vi "Main.vi"() -> ()   [LabVIEW 2014]
uses:
  Event_class/EventMsg.lvclass
  SubPanel/SubPanelModule.lvlib
panel:
  in  "Open Button":bool
  out "data":string
  in  "String":string
  in  "stop":bool
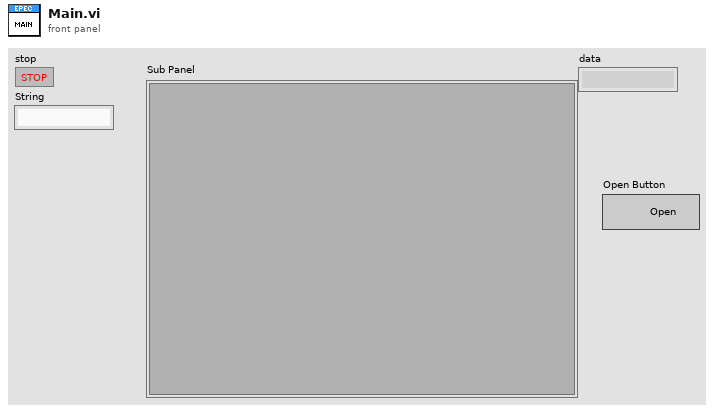
[diagram p1: front panel]
types:
  T1 = cluster{"EventClass":cluster{"object out":refnum<class "EventMsg.lvclass">}, "SubPanelData":cluster{"SubPanelPath":path, "SubPanelsVis":string[], "SubP_VIsPathList":path[], "VisRefs":refnum<vi>[]}}
  T2 = cluster{"object out":refnum<class "EventMsg.lvclass">}
  T3 = cluster{"SubPanelPath":path, "SubPanelsVis":string[], "SubP_VIsPathList":path[], "VisRefs":refnum<vi>[]}
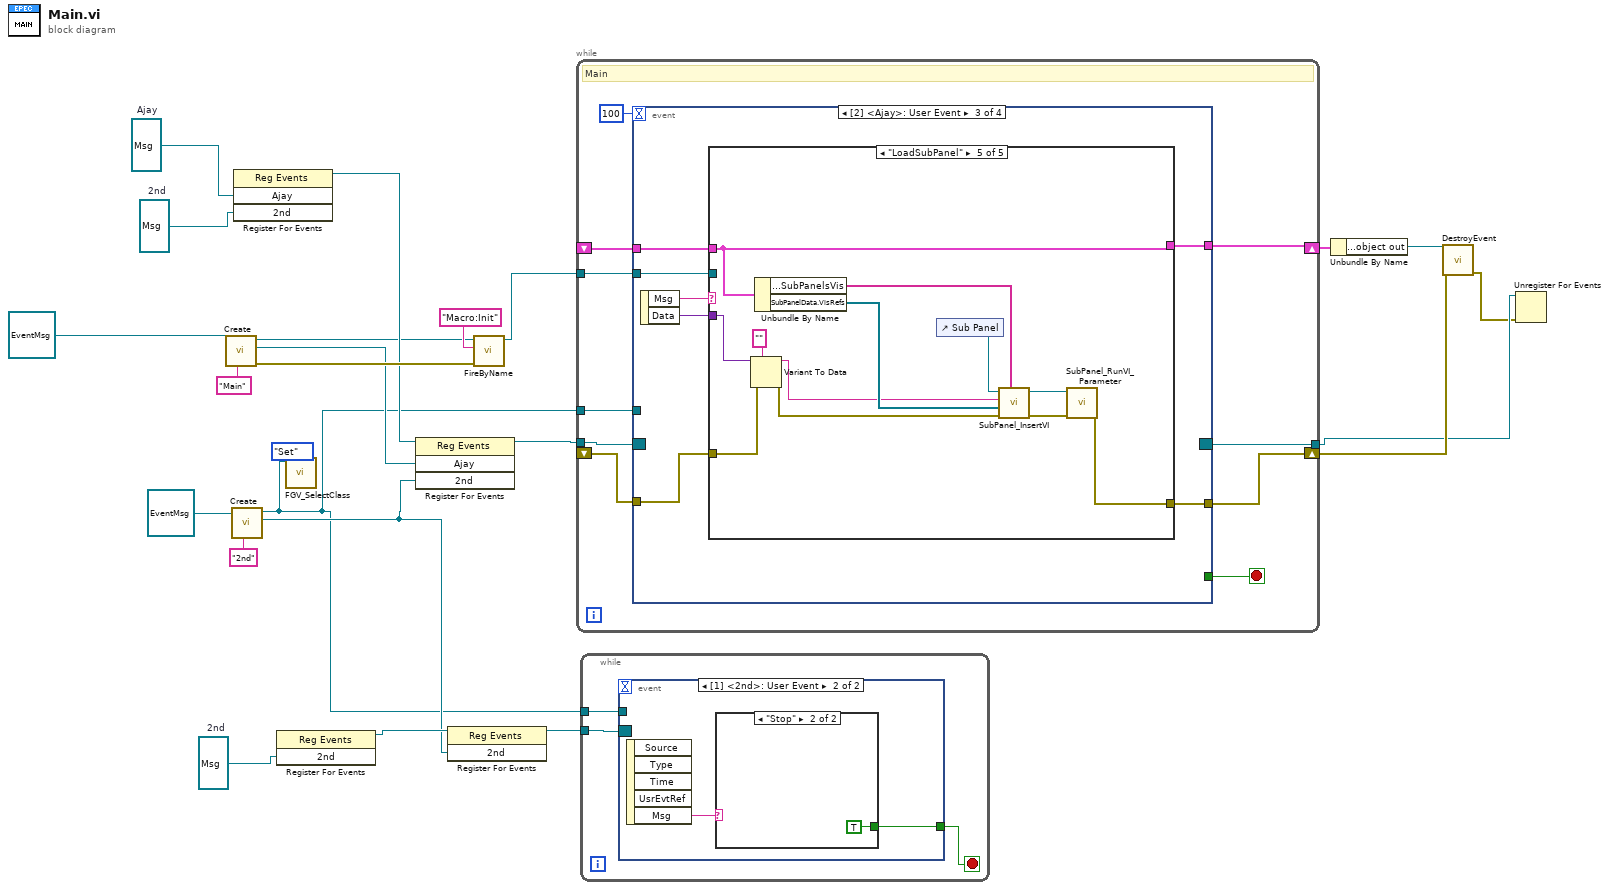
[diagram p0: block diagram]
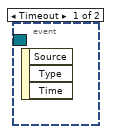
[diagram p2: hidden frame]
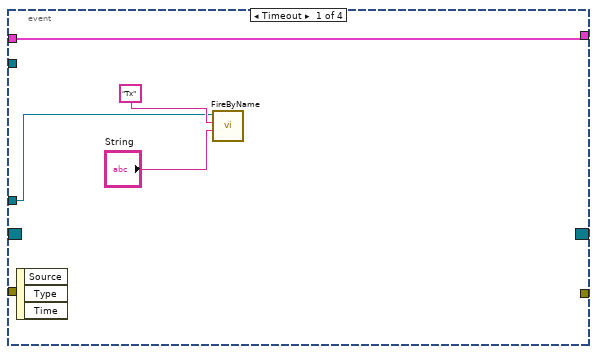
[diagram p4: hidden frame]
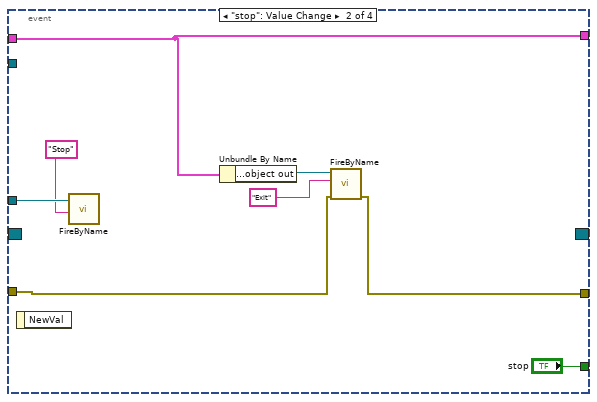
[diagram p5: hidden frame]
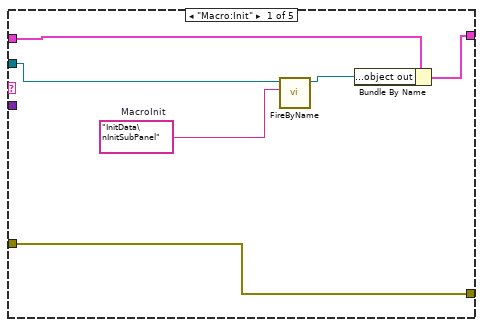
[diagram p6: hidden frame]
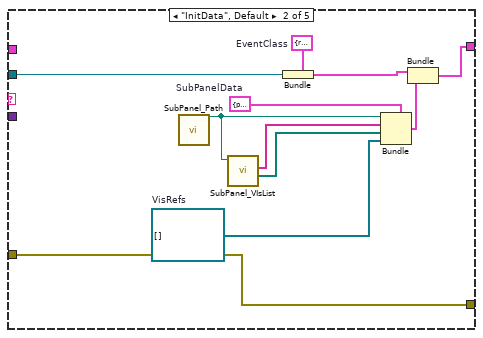
[diagram p7: hidden frame]
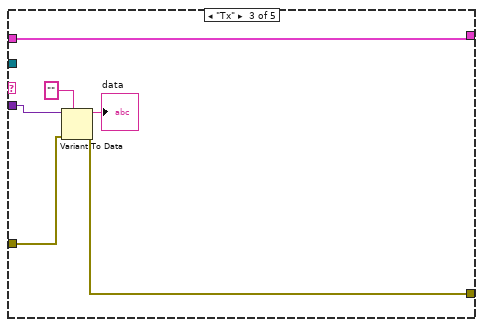
[diagram p8: hidden frame]
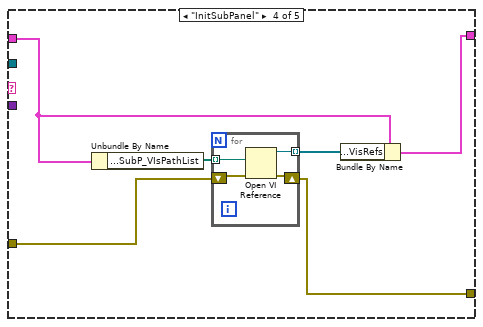
[diagram p9: hidden frame]
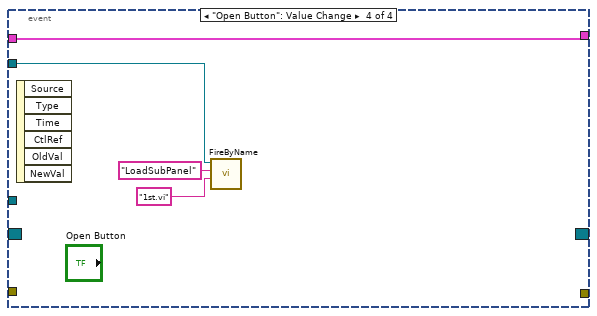
[diagram p10: hidden frame]
diagram:
  w9 = refnum<user-event> refnum  # 2nd
  w12 = refnum<user-event> refnum  # 2nd
  w17 = refnum<user-event> refnum  # Ajay
  n1 = call-dynamic "Create.vi"("Name"="Main", "object in"=refnum<class "EventMsg.lvclass"> refnum) -> ("error out"=w18:errorcluster, "user event out"=w15:refnum<user-event>, "object out"=w2:refnum<class "EventMsg.lvclass">)  [unwired: 7 in]
  n2 = call-dynamic "Create.vi"("Name"="2nd", "object in"=refnum<class "EventMsg.lvclass"> refnum) -> ("user event out"=w8:refnum<user-event>, "object out"=w1:refnum<class "EventMsg.lvclass">)  [unwired: 7 in, 1 out]
  n3 = register-events(w17, w12) -> (reference out=w16:refnum<event-registration>)  [unwired: 2 in, 1 out]
  n4 = register-events(w9) -> (reference out=w10:refnum<event-registration>)  [unwired: 2 in, 1 out]
  n5 = call "FGV_SelectClass.vi"("Action"=enum16{"Set", "Get"}."Set", "EventMsg.lvclass"=w1) -> ()  [unwired: 9 in, 1 out]
  n6 = register-events(reference=w16, w15, w8) -> (reference out=w14:refnum<event-registration>)  [unwired: 1 in, 1 out]
  n7 = register-events(reference=w10, w8) -> (reference out=w11:refnum<event-registration>)  [unwired: 1 in, 1 out]
  n8 = call-dynamic "FireByName.vi"("error in (no error)"=w18, "Msg"="Macro:Init", "object in"=w2) -> ("object out"=w22:refnum<class "EventMsg.lvclass">)  [unwired: 7 in, 1 out]
  n9 = while {
    shift-right: [w32] -> w19
    shift-left: _ -> [w33]
    shift-right: [w31] -> w21
    shift-left: _ -> [w30]
    tunnel: w22 -> [w29]
    tunnel: [w28] -> w5
    tunnel: w14 -> [w27]
    tunnel: w1 -> [w26]
    stop <- w34 stop-if-true
    # "Main"
    n10 = event shown="[2] <Ajay>: User Event" {
      selector: w27 -> [_ _ _ _]
      dyn-events: [_ _ _ _] -> w28
      timeout: 100 -> [_ _ _ _]
      tunnel: [_ "stop" _ _] -> w34
      tunnel: w33 -> [_ w43 w51 _]
      tunnel: [_ w42 w50 _] -> w32
      tunnel: [w38 w41 w49 w102] -> w31
      tunnel: w30 -> [w38 w41 w48 w102]
      tunnel: w29 -> [_ _ w47 w101]
      tunnel: w26 -> [w35 w40 _ _]
      event Timeout {
        n11 = event-data() -> ()  [unwired: 1 in, 3 out]
        n12 = call-dynamic "FireByName.vi"("Data"="String", "Msg"="Tx", "object in"=w35) -> ()  [unwired: 7 in, 2 out]
      }
      event "stop": Value Change {
        n13 = event-data() -> ()  [unwired: 1 in, 1 out]
        n14 = call-dynamic "FireByName.vi"("Msg"="Stop", "object in"=w40) -> ()  [unwired: 8 in, 2 out]
        n15 = Unbundle By Name(w41) -> ("EventClass.object out"=w45:refnum<class "EventMsg.lvclass">)
        n16 = call-dynamic "FireByName.vi"("error in (no error)"=w43, "Msg"="Exit", "object in"=w45) -> ("error out"=w42:errorcluster)  [unwired: 7 in, 1 out]
      }
      event User Event {
        n17 = event-data() -> ("Msg"=w52:string, "Data"=w53:variant)  [unwired: 1 in]
        n18 = case shown="\"LoadSubPanel\"" w52 {
          tunnel: w53 -> [_ _ w76 _ w91]
          tunnel: w51 -> [w55 w70 w73 w79 w88]
          tunnel: [w55 w70 w72 w78 w98] -> w50
          tunnel: [w58 w61 w71 w81 w93] -> w49
          tunnel: w48 -> [w59 _ w71 w80 w93]
          tunnel: w47 -> [w54 w64 _ _ _]
          frame "Macro:Init" {
            w56 = "InitData\nInitSubPanel"  # MacroInit
            n19 = call-dynamic "FireByName.vi"("Msg"=w56, "object in"=w54) -> ("object out"=w57:refnum<class "EventMsg.lvclass">)  [unwired: 8 in, 1 out]
            n20 = Bundle By Name(cluster=w59, "EventClass.object out"=w57) -> (w58:T1)
          }
          frame "InitData", Default {
            w65 = T2 {"object out"=refnum}  # EventClass
            w66 = T3 {"SubPanelPath"=path "", "SubPanelsVis"=[], "SubP_VIsPathList"=[], "VisRefs"=[]}  # SubPanelData
            w60 = refnum<vi>[] []  # VisRefs
            n21 = call "SubPanel_Path.vi"() -> ("SubPanelPath"=w69:path)  [unwired: 11 in]
            n22 = call "SubPanel_VIsList.vi"("SubPanelPath in"=w69) -> ("SubP_VIsPathList"=w67:path[], "SubPanelsVis"=w68:string[])  [unwired: 7 in, 2 out]
            n23 = Bundle(cluster=w65, "object out"=w64) -> (w63:T2)
            n24 = Bundle(cluster=w66, "SubPanelPath"=w69, "SubPanelsVis"=w68, "SubP_VIsPathList"=w67, "VisRefs"=w60) -> (w62:T3)
            n25 = Bundle("EventClass"=w63, "SubPanelData"=w62) -> (w61:T1)  [unwired: 1 in]
          }
          frame "Tx" {
            n26 = Variant To Data(error in=w73, type="", Variant=w76) -> (data=→"data":string, error out=w72:errorcluster)
          }
          frame "InitSubPanel" {
            n27 = Unbundle By Name(w80) -> ("SubPanelData.SubP_VIsPathList"=w82:path[])
            n28 = for {
              tunnel: w82 -> [w85] mode=indexing
              tunnel: [w86] -> w77 mode=indexing
              shift-right: [w83] -> w78
              shift-left: w79 -> [w84]
              n29 = Open VI Reference(vi path=w85, error in (no error)=w84) -> (vi reference=w86:refnum<vi>, error out=w83:errorcluster)  [unwired: 4 in]
            }
            n30 = Bundle By Name(cluster=w80, "SubPanelData.VisRefs"=w77) -> (w81:T1)
          }
          frame "LoadSubPanel" {
            n31 = Variant To Data(error in=w88, type="", Variant=w91) -> (data=w89:string, error out=w87:errorcluster)
            n32 = Unbundle By Name(w93) -> ("SubPanelData.SubPanelsVis"=w96:string[], "SubPanelData.VisRefs"=w92:refnum<vi>[])
            n33 = control-ref of="Sub Panel"() -> (w97:refnum<vi>)
            n34 = call "SubPanel_InsertVI.vi"("SubPanVI_Names"=w96, "error in (no error)"=w87, "SubPanRefs"=w92, "InsertVI_Name"=w89, "SubPanel in"=w97) -> ("error out"=w94:errorcluster, "InsertedVI"=w95:refnum<vi>)  [unwired: 5 in]
            n35 = call "SubPanel_RunVI_Parameter.vi"("error in (no error)"=w94, "VIref in"=w95) -> ("error out"=w98:errorcluster)  [unwired: 8 in, 1 out]
          }
        }
      }
      event "Open Button": Value Change {
        n36 = event-data() -> ()  [unwired: 1 in, 6 out]
        n37 = call-dynamic "FireByName.vi"("Data"="1st.vi" ("Msg"), "Msg"="LoadSubPanel", "object in"=w101) -> ()  [unwired: 7 in, 2 out]
      }
    }
  }
  n38 = while {
    tunnel: w1 -> [w103]
    tunnel: w11 -> [w104]
    stop <- w105 stop-if-true
    n39 = event shown="[1] <2nd>: User Event" {
      selector: w104 -> [_ _]
      dyn-events: _ -> [_ _]
      timeout: _ -> [_ _]
      tunnel: [_ w106] -> w105
      tunnel: w103 -> [_ _]
      event Timeout {
        n40 = event-data() -> ()  [unwired: 1 in, 3 out]
      }
      event User Event {
        n41 = event-data() -> ("Msg"=w107:string)  [unwired: 1 in, 4 out]
        n42 = case shown="\"Stop\"" w107 {
          tunnel: [_ TRUE] -> w106
          frame "False", Default {
          }
          frame "Stop" {
          }
        }
      }
    }
  }
  n43 = Unbundle By Name(w21) -> ("EventClass.object out"=w20:refnum<class "EventMsg.lvclass">)
  n44 = call-dynamic "DestroyEvent.vi"("error in (no error)"=w19, "object in"=w20) -> ("error out"=w4:errorcluster)  [unwired: 8 in, 1 out]
  n45 = Unregister For Events(event registration refnum=w5, error in=w4) -> ()  [unwired: 1 out]
